vi "WaveFormToString.vi"(7 "channelName":string, 11 "Waveform":waveform(dbl)) -> (3 "string":string)   [LabVIEW 2011]
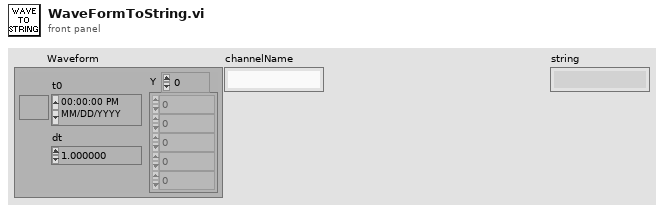
[diagram p1: front panel]
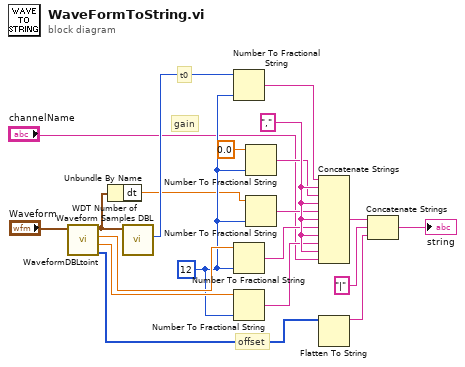
[diagram p0: block diagram]
diagram:
  w10 = i16 12 ("precision (6)")
  w15 = "," ("string")
  # "gain"
  # "offset"
  # "t0"
  n1 = call "WaveformDBLtoint.vi"("Waveform"="Waveform") -> ("32bit integer"=w18:i16[], "scale"=w20:dbl, "offset"=w19:dbl, "waveform out"=w2:waveform(dbl))  [unwired: 7 in]
  n2 = Unbundle By Name(w2) -> ("dt"=w1:dbl)
  n3 = call "WDT Number of Waveform Samples DBL.vi"("waveform in"=w2) -> ("number of samples"=w16:i32)  [unwired: 8 in, 2 out]
  n4 = Number To Fractional String(number=w16, precision (6)=w10) -> (F-format string=w6:string)  [unwired: 2 in]
  n5 = Number To Fractional String(number=w19, precision (6)=w10) -> (F-format string=w14:string)  [unwired: 2 in]
  n6 = Number To Fractional String(number=w20, precision (6)=w10) -> (F-format string=w9:string)  [unwired: 2 in]
  n7 = Number To Fractional String(number=0.0, precision (6)=w10) -> (F-format string=w7:string)  [unwired: 2 in]
  n8 = Number To Fractional String(number=w1, precision (6)=w10) -> (F-format string=w8:string)  [unwired: 2 in]
  n9 = Concatenate Strings(w6, w15, w7, w15, w8, w15, w14, w15, w9, w15, "channelName") -> (w11:string)
  n10 = Flatten To String(anything=w18) -> (data string=w13:string)  [unwired: 3 in, 2 out]
  n11 = Concatenate Strings(w11, "|" ("string"), w13) -> (→"string":string)
